vi "error database show.vi"() -> ()   [LabVIEW 2019]
uses:
  <vilib>/addons/database/Connection.llb/DB Tools Open Connec (String).vi
  <vilib>/addons/database/_DB Variant To Data/Database Variant To Data.xnode
  <vilib>/addons/database/NI_Database_API.lvlib
panel:
  out "error out":errorcluster
  in  "Close Square":bool
  in  "Delete Button":bool
  in  "Refresh Button":bool
  out "ERROR  TABLE":string[][](table)
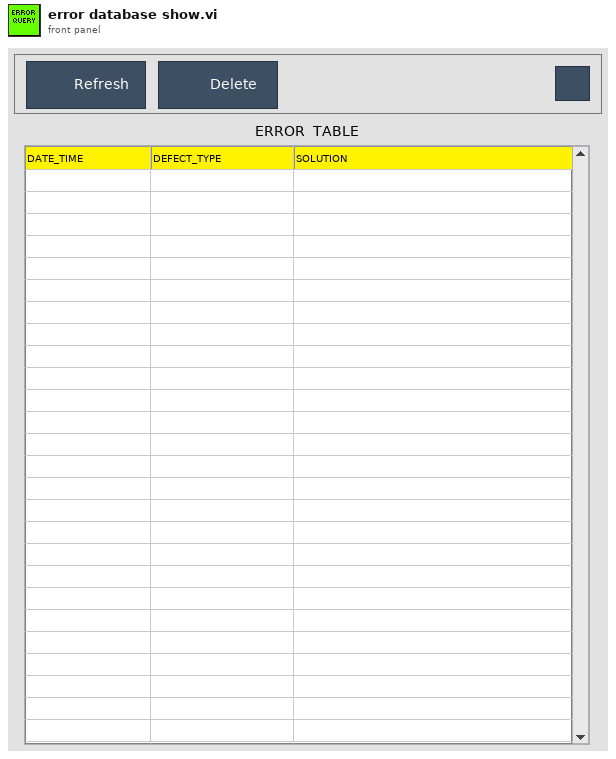
[diagram p1: front panel]
types:
  T1 = typedef "NI_Database_API.lvlib/Conn ObjectReference.ctl" = refnum<k1>
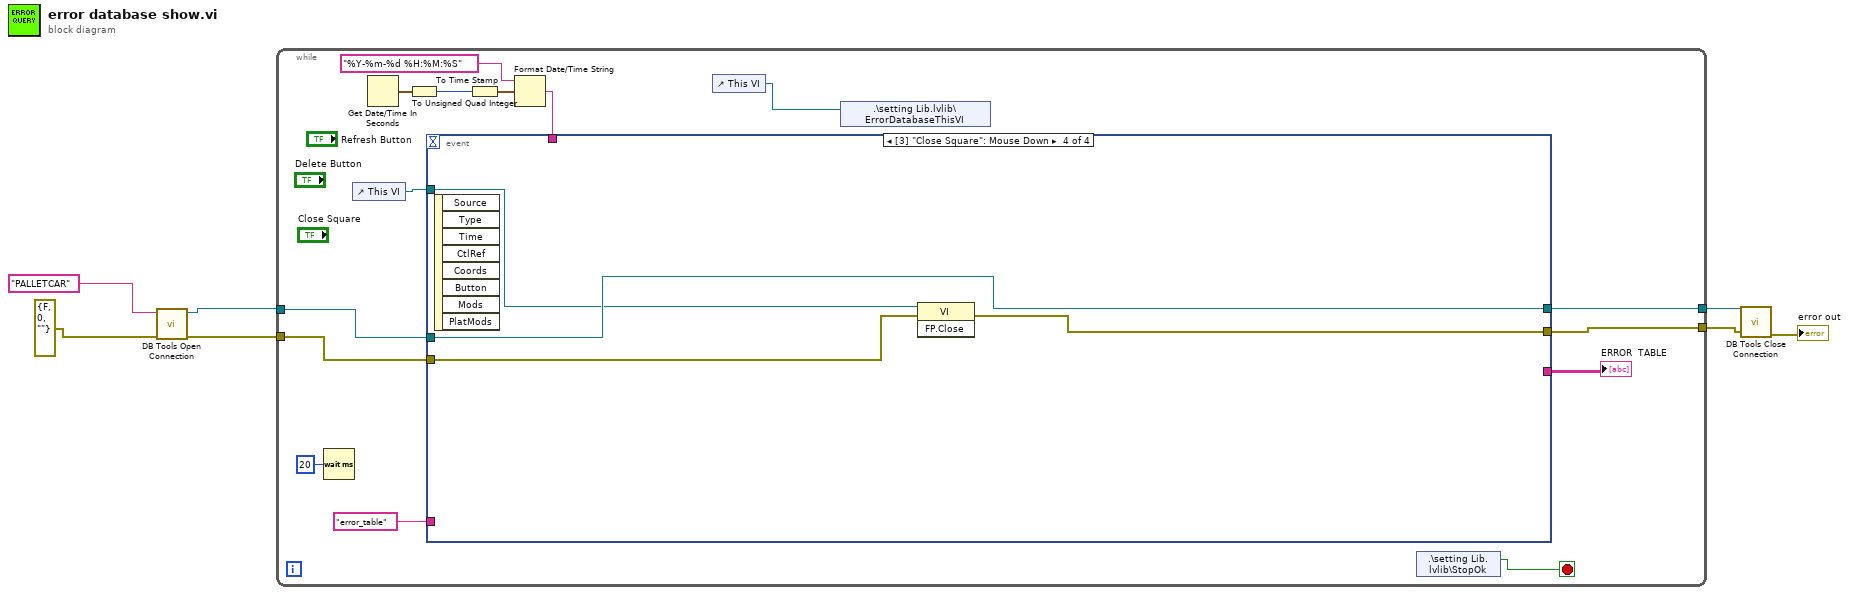
[diagram p0: block diagram]
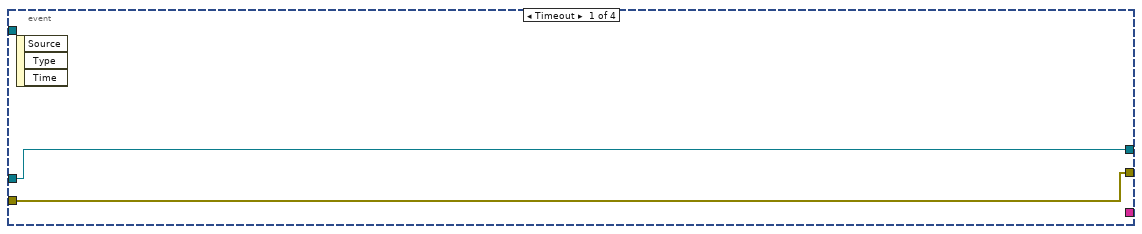
[diagram p2: hidden frame]
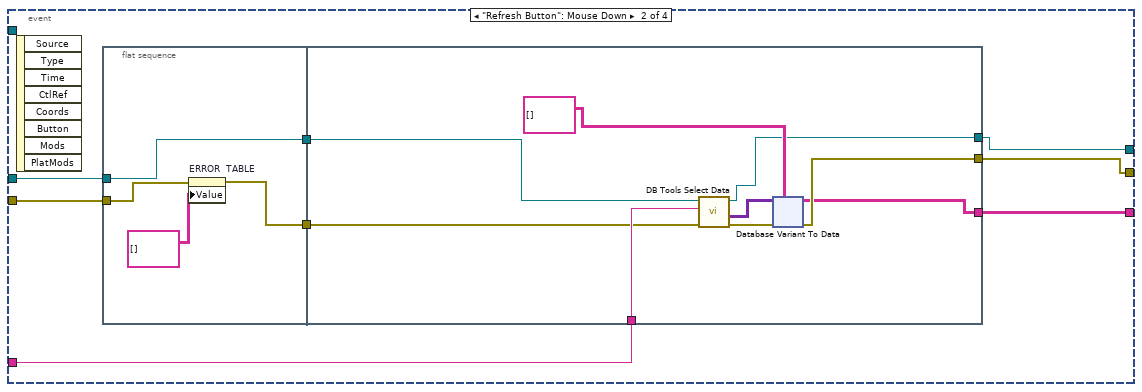
[diagram p3: hidden frame]
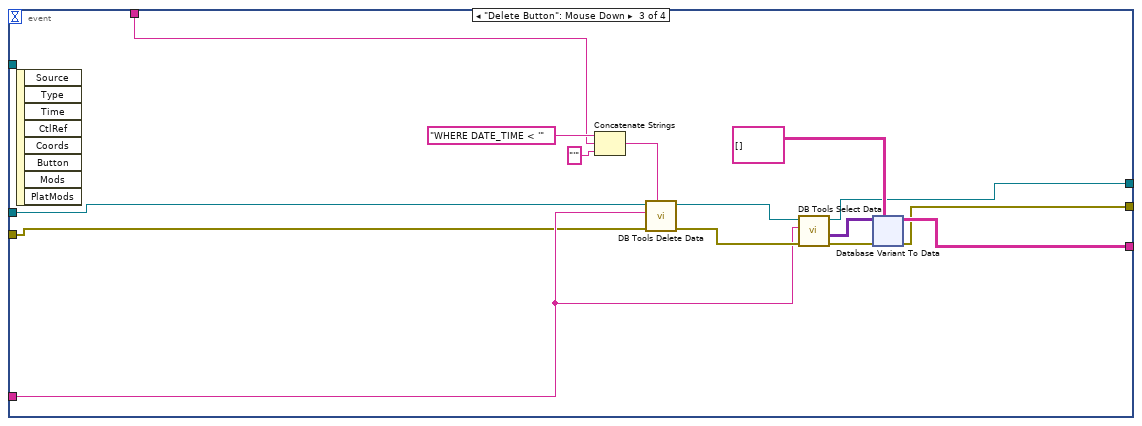
[diagram p4: hidden frame]
diagram:
  n1 = call-poly <vilib>:"DB Tools Open Connection.vi"("error in (no error)"=errorcluster {"status"=FALSE, "code"=0, "source"=""}, "connection information"="PALLETCAR" ("database name")) -> ("error out"=w4:errorcluster, "connection reference"=w5:T1)  [unwired: 6 in]
  n2 = while {
    tunnel: w5 -> [w14]
    tunnel: w4 -> [w13]
    tunnel: [w12] -> w3
    tunnel: [w11] -> w2
    stop <- w9 stop-if-true
    n3 = Wait (ms)(milliseconds to wait=u32 20) -> ()  [unwired: 1 out]
    n4 = control-ref of="This VI"() -> (w10:refnum<vi>)
    n5 = Get Date/Time In Seconds() -> (seconds since 1Jan1904=w18:timestamp)
    n6 = To Unsigned Quad Integer(1:w18) -> (0:w19:u64)
    n7 = To Time Stamp(1:w19) -> (0:w20:timestamp)
    n8 = Format Date/Time String(time format string (%c)="%Y-%m-%d %H:%M:%S", seconds (now)=w20) -> (date/time string=w17:string)  [unwired: 1 in]
    n9 = event shown="[3] \"Close Square\": Mouse Down" {
      selector: _ -> [_ _ _ _]
      dyn-events: _ -> [_ _ _ _]
      timeout: _ -> [_ _ _ _]
      tunnel: "error_table" ("table") -> [_ w32 w97 _]
      tunnel: [w23 w25 w90 w152] -> w12
      tunnel: w17 -> [_ _ w102 _]
      tunnel: [_ w31 w95 _] -> w15
      tunnel: w14 -> [w24 w29 w93 w151]
      tunnel: w13 -> [w23 w28 w92 w150]
      tunnel: [w24 w26 w91 w151] -> w11
      tunnel: w10 -> [_ _ _ w149]
      event Timeout {
        n10 = event-data() -> ()  [unwired: 1 in, 3 out]
      }
      event "Refresh Button": Mouse Down {
        n11 = event-data() -> ()  [unwired: 1 in, 8 out]
        n12 = flat-sequence {
          tunnel: [w35] -> w30
          tunnel: w29 -> [w35]
          tunnel: w28 -> [w34]
          tunnel: [w33] -> w27
          tunnel: [w42] -> w26
          tunnel: [w41] -> w25
          tunnel: w32 -> [w40]
          tunnel: [w39] -> w31
          tunnel: w30 -> [w38]
          tunnel: w27 -> [w37]
          frame #0 {
            n13 = property on="ERROR  TABLE" class="Tbl (strict)"(error in=w34, "Value"=string[][] [] ("DEFECTS  TABLE")) -> (error out=w33:errorcluster)  [unwired: 1 in, 1 out]
          }
          frame #1 {
            n14 = call <vilib>:"DB Tools Select Data.vi"("error in (no error)"=w37, "table"=w40, "connection reference"=w38) -> ("error out"=w44:errorcluster, "data"=w45:variant[][], "connection reference out"=w42:T1)  [unwired: 3 in]
            n15 = xnode "Database Variant To Data"("database variant"=w45, "error in (no error)"=w44, "type"=string[][] []) -> ("data"=w39:string[][], "error out"=w41:errorcluster)
          }
        }
      }
      event "Delete Button": Mouse Down {
        n16 = event-data() -> ()  [unwired: 1 in, 8 out]
        n17 = Concatenate Strings("WHERE DATE_TIME < '" ("condition"), w102, "'" ("condition")) -> (w96:string)
        n18 = call <vilib>:"DB Tools Delete Data.vi"("condition"=w96, "error in (no error)"=w92, "table"=w97, "connection reference"=w93) -> ("error out"=w98:errorcluster, "connection reference out"=w99:T1)  [unwired: 6 in]
        n19 = call <vilib>:"DB Tools Select Data.vi"("error in (no error)"=w98, "table"=w97, "connection reference"=w99) -> ("error out"=w100:errorcluster, "data"=w101:variant[][], "connection reference out"=w91:T1)  [unwired: 3 in]
        n20 = xnode "Database Variant To Data"("database variant"=w101, "error in (no error)"=w100, "type"=string[][] []) -> ("data"=w95:string[][], "error out"=w90:errorcluster)
      }
      event "Close Square": Mouse Down {
        n21 = event-data() -> ()  [unwired: 1 in, 8 out]
        n22 = invoke class="VI" method="FP.Close"(reference=w149, error in=w150) -> (error out=w152:errorcluster)  [unwired: 1 in, 2 out]
      }
    }
    "ERROR  TABLE" <- w15
    n23 = control-ref of="This VI"() -> (w8:refnum<vi>)
    n24 = shared-variable ".\\setting Lib.lvlib\\ErrorDatabaseThisVI"(w8) -> ()  [unwired: 1 in, 1 out]
    n25 = shared-variable ".\\setting Lib.lvlib\\StopOk"() -> (w9:bool)  [unwired: 1 in, 1 out]
  }
  n26 = call <vilib>:"DB Tools Close Connection.vi"("error in (no error)"=w3, "connection reference"=w2) -> ("error out"=→"error out":errorcluster)  [unwired: 5 in]
